vi "Pre-Actor.vi"(8 "error in":errorcluster, 11 "MLTFNC in":refnum<class "MLTFNC.lvclass">) -> (0 "error out":errorcluster, 3 "MLTFNC out":refnum<class "MLTFNC.lvclass">)   [LabVIEW 2019, in "MLTFNC.lvlib" / "MLTFNC.lvclass"]
doc: "This override VI is to provide the means for children classes to perform application specific post launch initialization functions that must be performed *prior* to calling the actor. \n\n***DO NOT USE THE CHECK FOR FAULT ROUTINE HERE***"
uses:
  Library/MLTFNC.lvclass
  Library/MLTFNC.lvclass/MLTFNC.ctl
  builds/Instruments/Instruments.lvlibp/Library/Instruments.lvclass
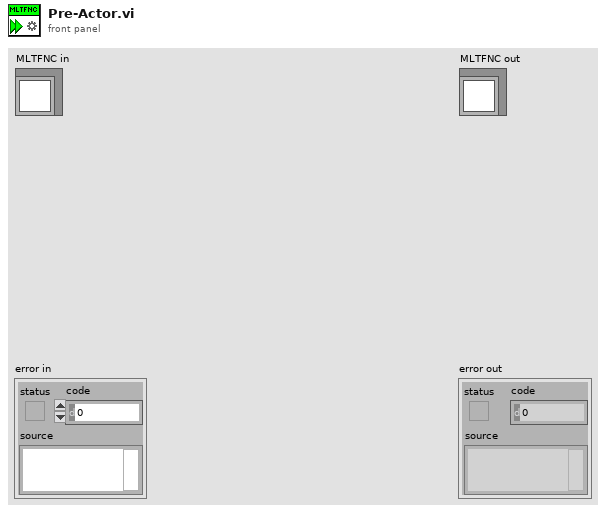
[diagram p1: front panel]
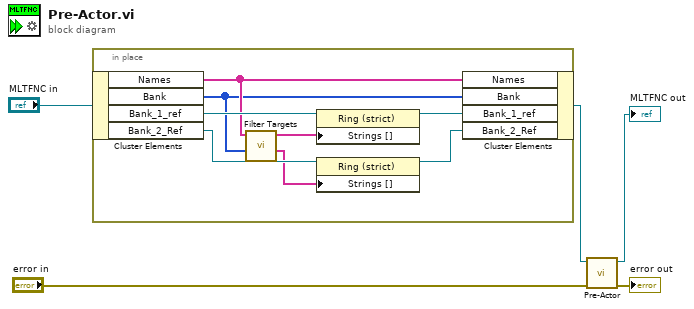
[diagram p0: block diagram]
diagram:
  n1 = in-place {
    n2 = in-place-cluster #1("MLTFNC in") -> ("Names"=w9:string[], "Bank"=w6:u32[], "Bank_1_ref"=w13:refnum<vi>, "Bank_2_Ref"=w12:refnum<vi>)
    n3 = call "Filter Targets.vi"("Bank"=w6, "Names"=w9) -> ("Bank 2"=w7:string[], "Bank 1"=w8:string[])  [unwired: 8 in]
    n4 = property class="Ring (strict)"(reference=w13, "Strings []"=w8) -> (reference out=w10:refnum<vi>)  [unwired: 1 in, 1 out]
    n5 = property class="Ring (strict)"(reference=w12, "Strings []"=w7) -> (reference out=w11:refnum<vi>)  [unwired: 1 in, 1 out]
    n6 = in-place-cluster #1("Names"=w9, "Bank"=w6, "Bank_1_ref"=w10, "Bank_2_Ref"=w11) -> (w2:refnum<class "MLTFNC.lvclass">)
  }
  n7 = call-parent "Pre-Actor.vi"("error in (no error)"="error in", "Instruments in"=w2) -> ("error out"=→"error out":errorcluster, "Instruments out"=→"MLTFNC out":refnum<class "MLTFNC.lvclass">)  [unwired: 8 in]
